vi "Main.vi"(8 "error in":errorcluster, 11 "Application Manager in":refnum<class "Application Manager.lvclass">) -> (0 "error out":errorcluster, 3 "Application Manager out":refnum<class "Application Manager.lvclass">)   [LabVIEW 2017, in "Application Manager.lvclass"]
doc: "The <b>Queued Message Handler</b> of the Worker that owns this VI."
uses:
  Application Manager.lvclass
  Buttons/Settings.ctl
  FP Refs.ctl
  <vilib>/Utility/miscctls.llb/LVPointTypeDef.ctl
  Application Manager.lvclass/Application Manager.ctl
  <vilib>/addons/_Workers/Library/Classes/Message/Priority.ctl
  Initialization Data.ctl
  Response Cases.ctl
  <vilib>/addons/_Workers/Library/Case Label.ctl
  rsp_Start Shutdown.ctl
  rql_RCM Show Message Log.ctl
  Tree Right Click Menu Data.ctl
  <vilib>/Utility/miscctls.llb/LVPoint32TypeDef.ctl
  rql_RCM Show Front Panel.ctl
  rql_RCM Show Block Diagram.ctl
  rql_RCM Send Start Exiting Request.ctl
  rql_RCM Filter as Enque Worker.ctl
  rql_RCM Filter as Deque Worker.ctl
  rwr_Get Shutdown Data Reply.ctl
  <vilib>/Utility/miscctls.llb/LVRectTypeDef.ctl
  rqp_Display User Message.ctl
  rqp_Show Front Panel.ctl
  <vilib>/Platform/browser.llb/Open URL in Default Browser (string).vi
  <vilib>/addons/_Workers/Library/Workers.lvlib
  <vilib>/addons/_Workers/Library/Classes/Message/Message.lvclass
panel:
  in  "settings":T1
  in  "ClearDisconnected":bool
  out "Message":string="Error : Port already in use"
  in  "Tree":string(tree)
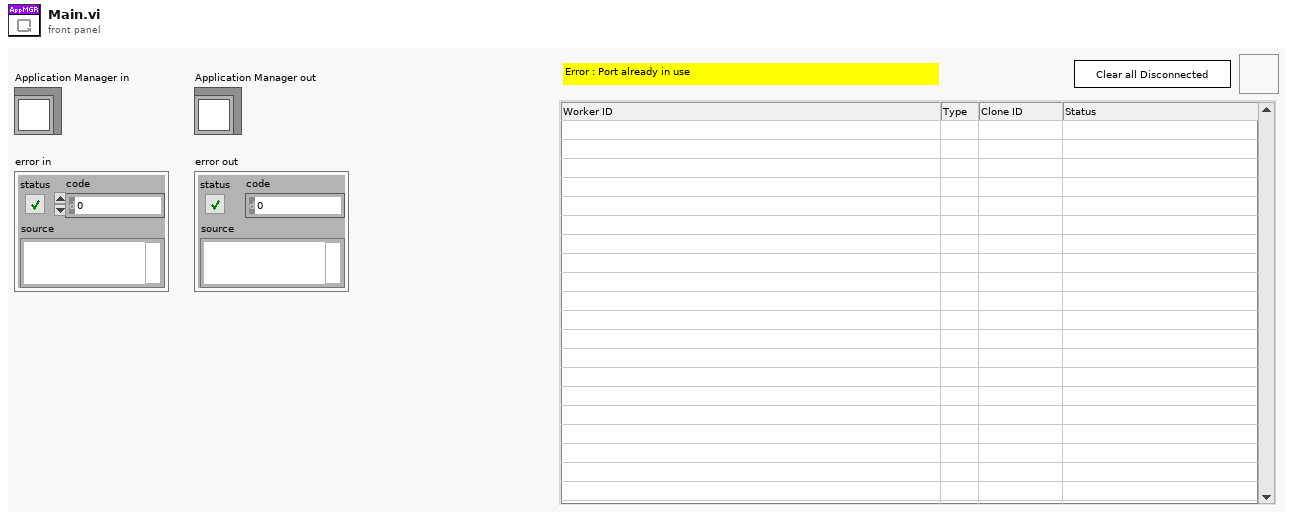
[diagram p1: front panel]
types:
  T1 = typedef "Settings.ctl" = bool
  T2 = typedef "LVPointTypeDef.ctl" = cluster{"Horizontal":i16, "Vertical":i16}
  T3 = typedef "Application Manager.lvclass/FP Refs.ctl" = cluster{"Message.Ref":refnum<vi>, "ClearDiscon.Ref":refnum<vi>, "Settings.Ref":refnum<vi>, "Tree.Ref":refnum<vi>}
  T4 = typedef "imagedata.ctl" = cluster{"image type":i32, "image depth":i32, "image":u8[], "mask":u8[], "colors":u32[], "Rectangle":cluster{"left":i16, "top":i16, "right":i16, "bottom":i16}}
  T5 = typedef "Application Manager.lvclass/Initialization Data.ctl" = cluster{"Response Cases":T6}
  T6 = typedef "Application Manager.lvclass/Response Cases.ctl" = cluster{"Show Settings Dialog":T7, "Start Shutdown":T7, "Show Message Log":T7, "New Head Worker Added":T7, "Show Worker Front Panel":T7, "Show Worker Block Diagram":T7, "Send Start Exiting Request":T7, "Filter as Enque Worker":T7, "Filter as Deque Worker":T7, "Go to MHL Case - Response":T7}
  T7 = typedef "Workers.lvlib/Case Label.ctl" = string
  T8 = typedef "Application Manager.lvclass/rsp_Start Shutdown.ctl" = cluster{"Monitor":u16}
  T9 = typedef "Workers.lvlib/Message.lvclass/Priority.ctl" = enum16{"Low", "Normal", "High"}
  T10 = typedef "Application Manager.lvclass/rql_RCM Show Message Log.ctl" = cluster{"Tree RCM Data":T11}
  T11 = typedef "Application Manager.lvclass/Tree Right Click Menu Data.ctl" = cluster{"CtlRef":refnum<vi>, "Coords":T12}
  T12 = typedef "LVPoint32TypeDef.ctl" = cluster{"Horizontal":i32, "Vertical":i32}
  T13 = typedef "Application Manager.lvclass/rql_RCM Show Front Panel.ctl" = cluster{"Tree RCM Data":T11}
  T14 = typedef "Application Manager.lvclass/rql_RCM Show Block Diagram.ctl" = cluster{"Tree RCM Data":T11}
  T15 = typedef "Application Manager.lvclass/rql_RCM Send Start Exiting Request.ctl" = cluster{"Tree RCM Data":T11}
  T16 = typedef "Application Manager.lvclass/rql_RCM Filter as Enque Worker.ctl" = cluster{"Tree RCM Data":T11}
  T17 = typedef "Application Manager.lvclass/rql_RCM Filter as Deque Worker.ctl" = cluster{"Tree RCM Data":T11}
  T18 = typedef "Application Manager.lvclass/rwr_Get Shutdown Data Reply.ctl" = cluster{"Window Bounds":T19, "Monitor":u16, "FP.State":enum32{"Invalid", "Standard", "Closed", "Hidden", "Minimized", "Maximized"}, "Column Widths":u32[]}
  T19 = typedef "LVRectTypeDef.ctl" = cluster{"Left":i16, "Top":i16, "Right":i16, "Bottom":i16}
  T20 = typedef "Application Manager.lvclass/rqp_Display User Message.ctl" = cluster{"Message":string, "BG Color":u32}
  T21 = typedef "Application Manager.lvclass/rqp_Show Front Panel.ctl" = cluster{"String":string}
  T22 = enum32{"Invalid", "Standard", "Closed", "Hidden", "Minimized", "Maximized"}
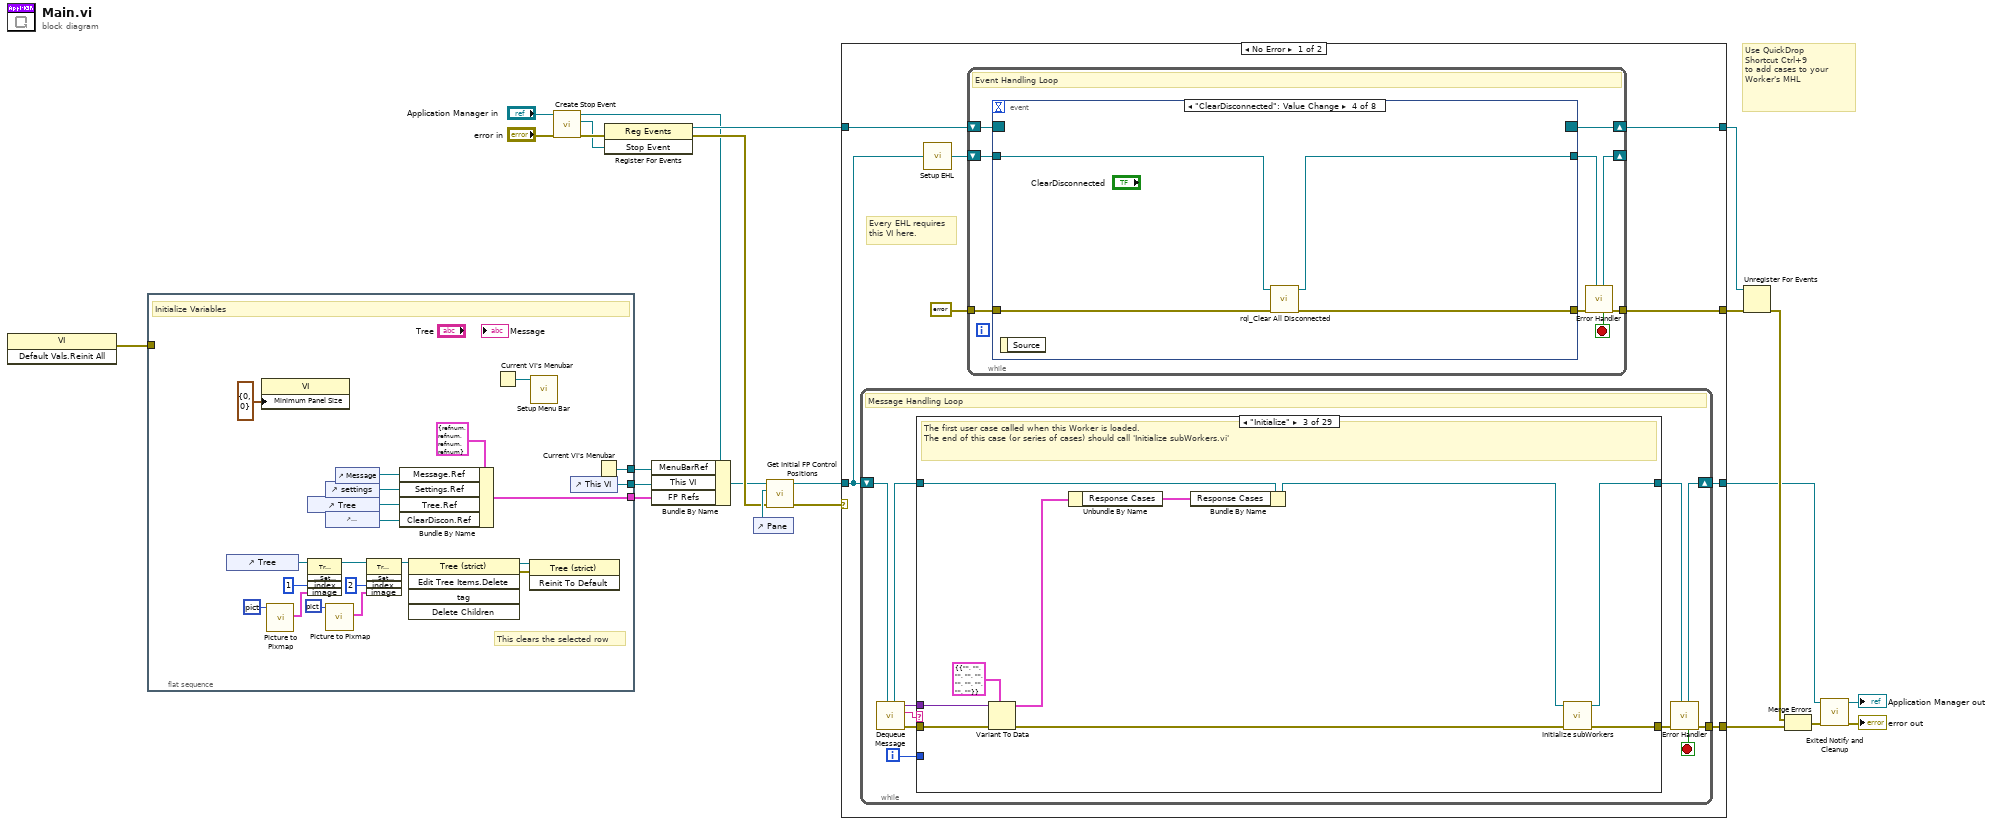
[diagram p0: block diagram]
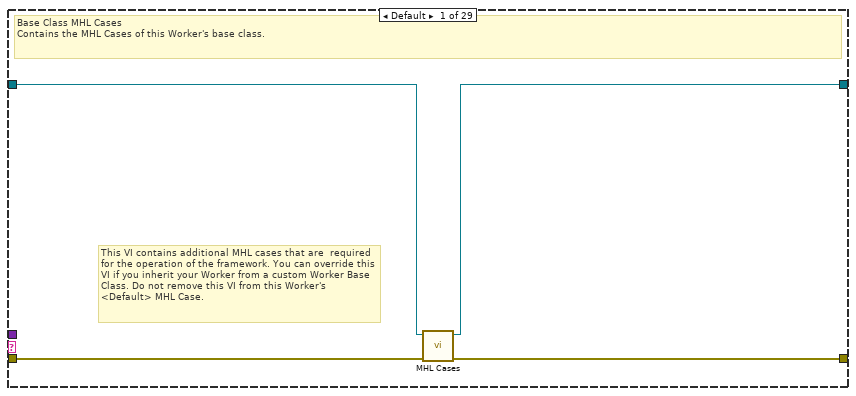
[diagram p2: hidden frame]
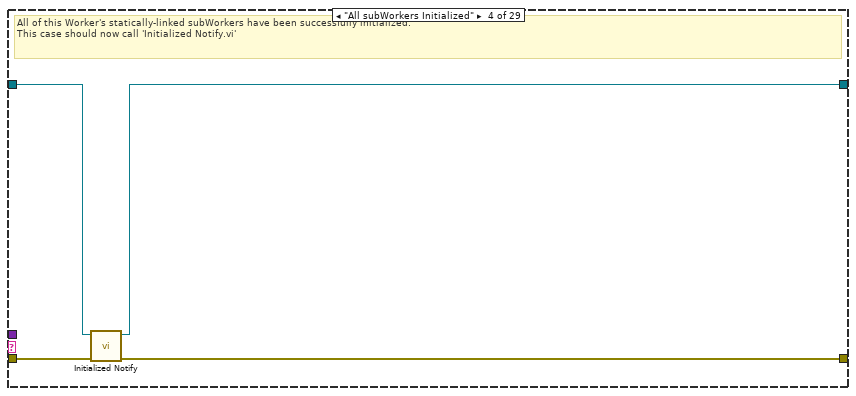
[diagram p4: hidden frame]
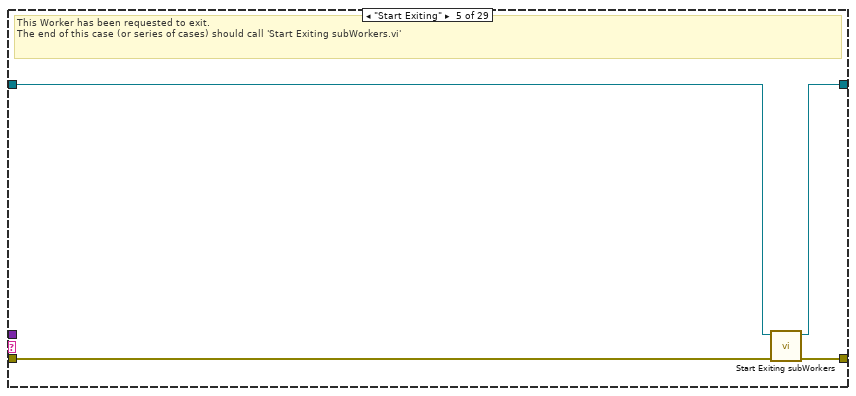
[diagram p5: hidden frame]
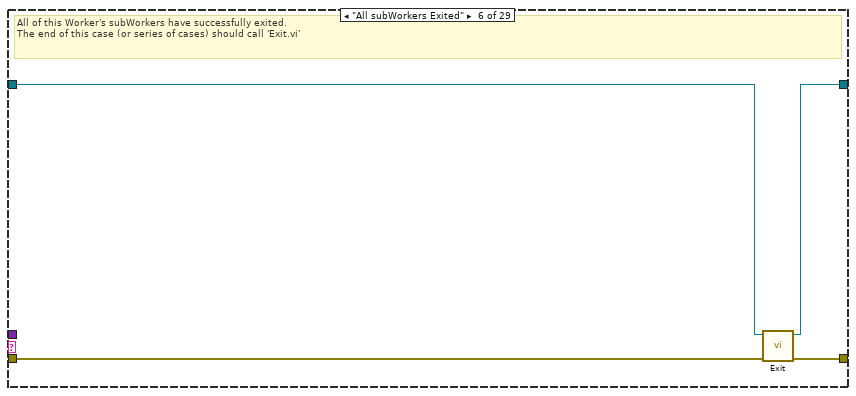
[diagram p6: hidden frame]
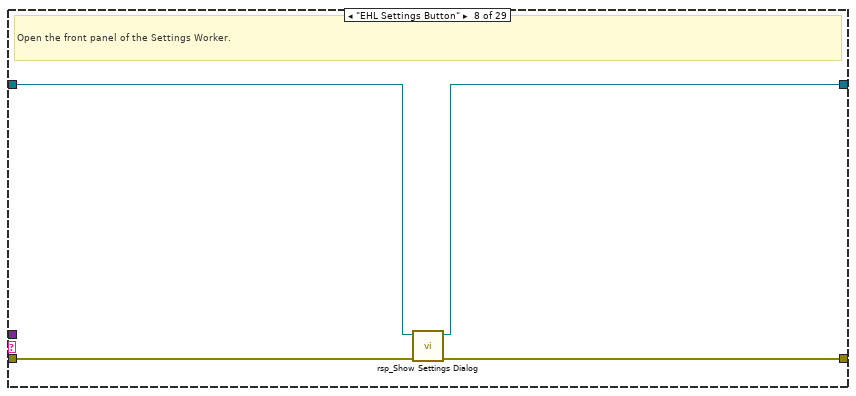
[diagram p8: hidden frame]
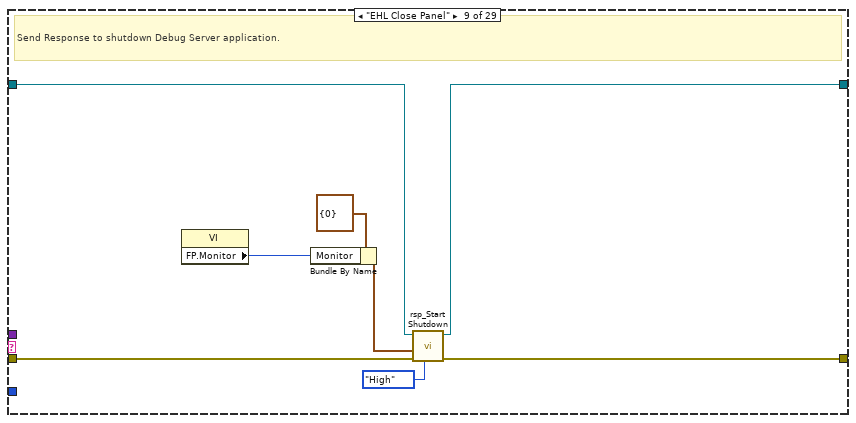
[diagram p9: hidden frame]
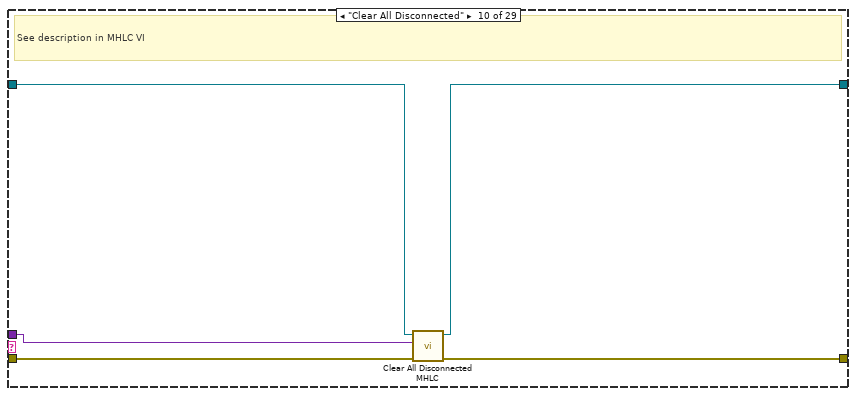
[diagram p10: hidden frame]
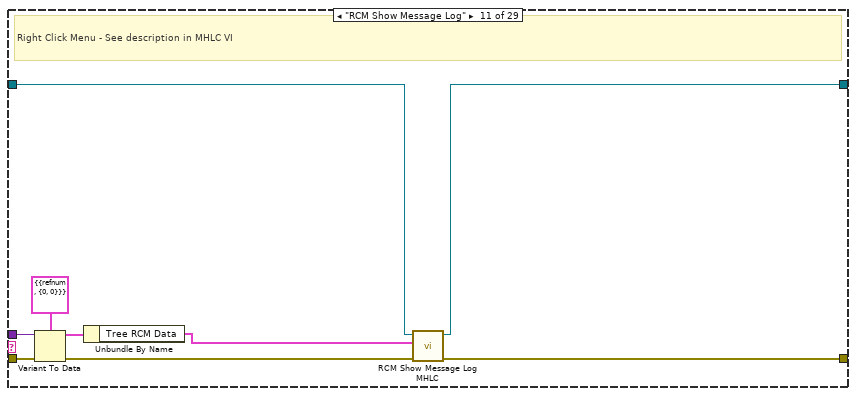
[diagram p11: hidden frame]
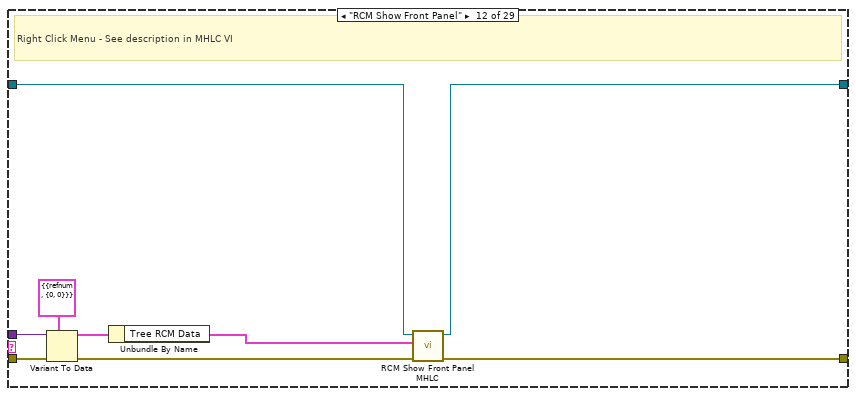
[diagram p12: hidden frame]
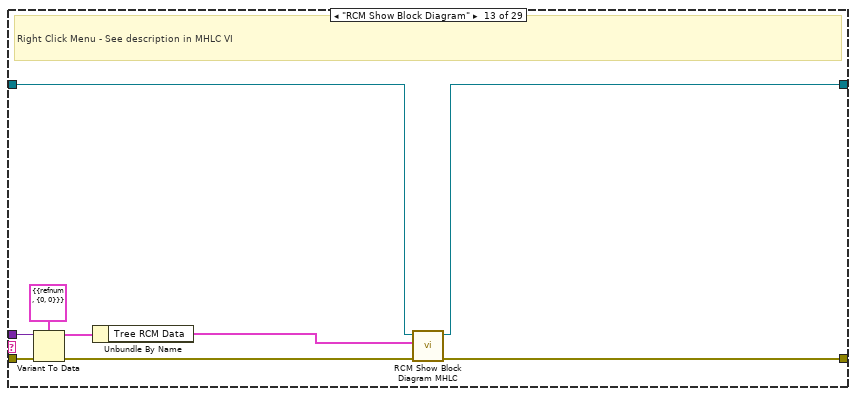
[diagram p13: hidden frame]
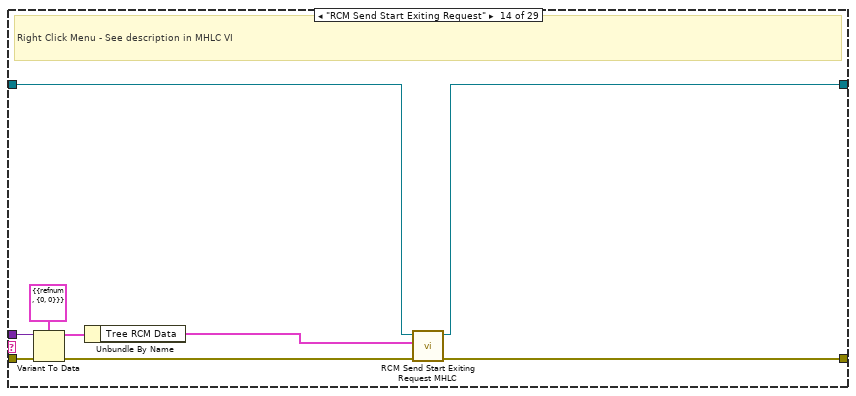
[diagram p14: hidden frame]
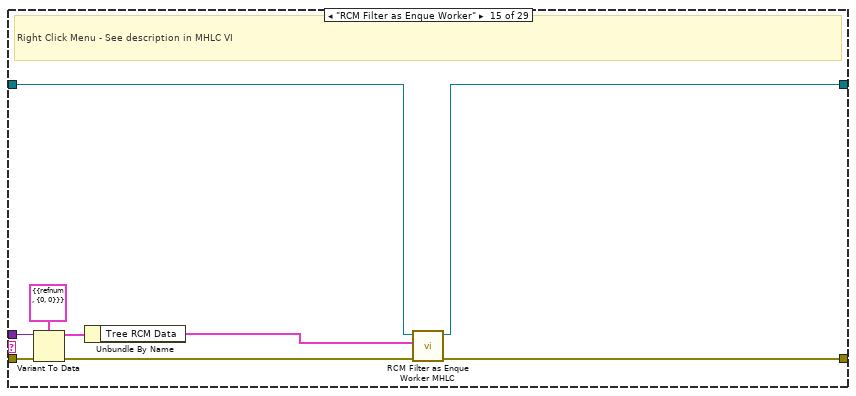
[diagram p15: hidden frame]
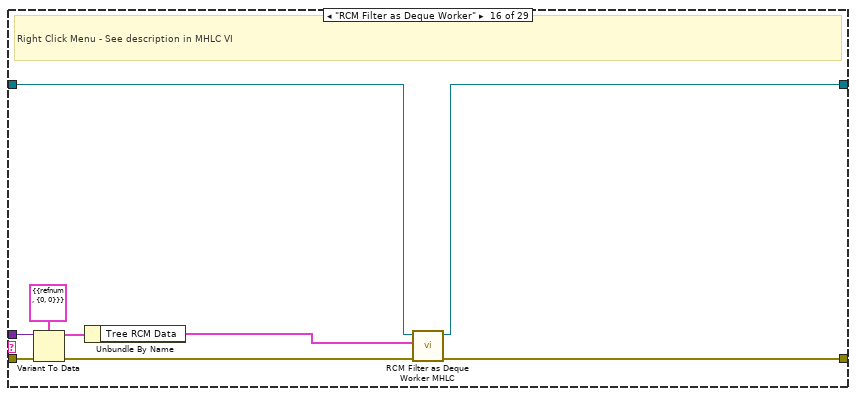
[diagram p16: hidden frame]
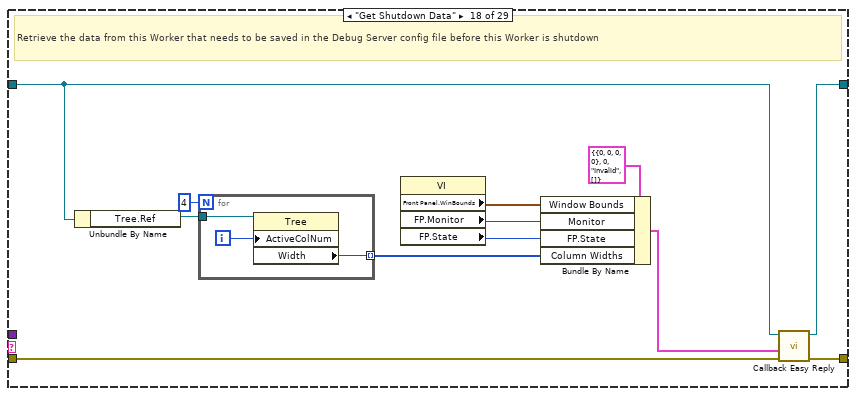
[diagram p18: hidden frame]
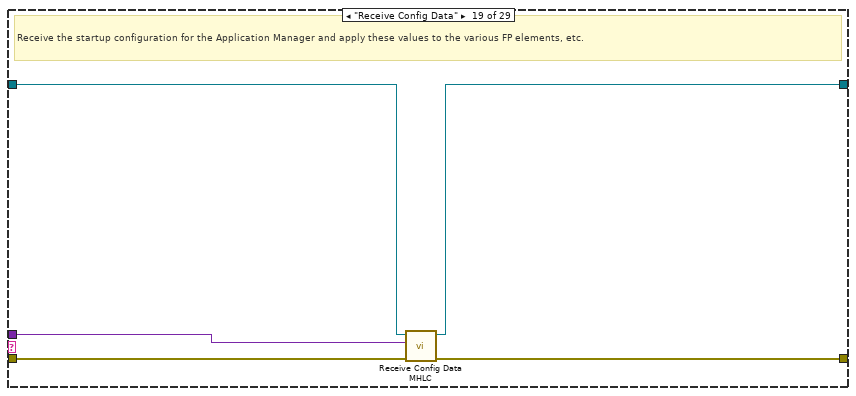
[diagram p19: hidden frame]
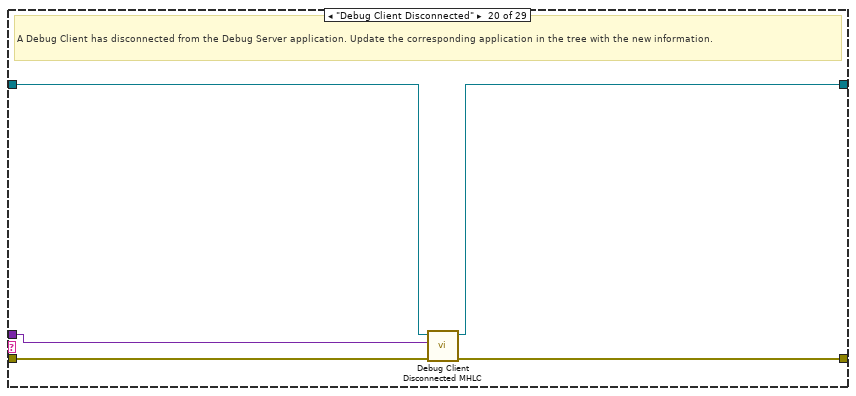
[diagram p20: hidden frame]
diagram:
  # "Use QuickDrop\nShortcut Ctrl+9\nto add cases to your\nWorker's MHL"
  n1 = invoke class="VI" method="Default Vals.Reinit All"() -> (error out=w8:errorcluster)  [unwired: 3 in, 2 out]
  n2 = flat-sequence {
    tunnel: w8 -> [_]
    tunnel: [w27] -> w5
    tunnel: [w26] -> w4
    tunnel: [w25] -> w3
    frame #0 {
      # "This clears the selected row"
      # "Initialize Variables"
      n3 = control-ref of="Tree"() -> (w33:refnum<vi>)
      n4 = property class="VI"("Minimum Panel Size"=T2 {"Horizontal"=0, "Vertical"=0} ("Front Panel Window:Minimum Size")) -> ()  [unwired: 2 in, 2 out]
      n5 = call <vilib>:"Picture to Pixmap.vi"("picture"=picture bytes[273] ("new picture")) -> ("image data"=w37:T4)  [unwired: 9 in, 1 out]
      n6 = control-ref of="Tree"() -> (w41:refnum<vi>)
      n7 = invoke on="Invoke Node" class="Tree (strict)" method="Custom Item Symbols.Set Symbol"(reference=w33, "index"=1 ("Index"), "image"=w37) -> (reference out=w38:refnum<vi>)  [unwired: 2 in, 4 out]
      n8 = control-ref of="settings"() -> (w28:refnum<vi>)
      n9 = control-ref of="ClearDisconnected"() -> (w42:refnum<vi>)
      n10 = call <vilib>:"Picture to Pixmap.vi"("picture"=picture bytes[273] ("new picture 2")) -> ("image data"=w35:T4)  [unwired: 9 in, 1 out]
      n11 = control-ref of="Message"() -> (w43:refnum<vi>)
      n12 = invoke on="Invoke Node" class="Tree (strict)" method="Custom Item Symbols.Set Symbol"(reference=w38, "index"=2 ("Index"), "image"=w35) -> (reference out=w30:refnum<vi>)  [unwired: 2 in, 4 out]
      n13 = Bundle By Name(cluster=T3 {"Message.Ref"=refnum, "ClearDiscon.Ref"=refnum, "Settings.Ref"=refnum, "Tree.Ref"=refnum} ("Data"), "Message.Ref"=w43, "Settings.Ref"=w28, "Tree.Ref"=w41, "ClearDiscon.Ref"=w42) -> (w25:T3)
      n14 = invoke class="Tree (strict)" method="Edit Tree Items.Delete"(reference=w30) -> (reference out=w32:refnum<vi>, error out=w31:errorcluster)  [unwired: 4 in, 3 out]
      n15 = Current VI's Menubar() -> (w24:refnum<k9>)
      n16 = invoke class="Tree (strict)" method="Reinit To Default"(reference=w32, error in=w31) -> ()  [unwired: 1 in, 3 out]
      n17 = call "Setup Menu Bar.vi"("menu reference"=w24) -> ()  [unwired: 10 in, 1 out]
      n18 = control-ref of="This VI"() -> (w26:refnum<vi>)
      n19 = Current VI's Menubar() -> (w27:refnum<k9>)
    }
  }
  n20 = call-dynamic "Create Stop Event.vi"("error in"="error in", "Worker"="Application Manager in") -> ("error out"=w18:errorcluster, "Stop Event"=w15:refnum<user-event>, "Worker out"=w6:refnum<class "Application Manager.lvclass">)  [unwired: 7 in]
  n21 = register-events(error in=w18, w15) -> (reference out=w17:refnum<event-registration>, error out=w9:errorcluster)  [unwired: 1 in]
  n22 = Bundle By Name(cluster=w6, "MenuBarRef"=w5, "This VI"=w4, "FP Refs"=w3) -> (w7:refnum<class "Application Manager.lvclass">)
  n23 = control-ref of="Pane"() -> (w10:refnum<vi>)
  n24 = call "Get Initial FP Control Positions.vi"("error in (no error)"=w9, "Pane"=w10, "AppMgr in"=w7) -> ("error out"=w2:errorcluster, "AppMgr out"=w1:refnum<class "Application Manager.lvclass">)  [unwired: 7 in]
  n25 = case shown="No Error" w2 {
    tunnel: w1 -> [w47 w309]
    tunnel: [w45 w310] -> w16
    tunnel: w17 -> [w52 w311]
    tunnel: [w49 w312] -> w22
    tunnel: [w51 w311] -> w21
    tunnel: [w46 w308] -> w19
    selector: w2 -> [_ w312]
    frame No Error {
      # "Every EHL requires\nthis VI here."
      n26 = while {
        shift-right: [w61] -> w46
        shift-left: w47 -> [w63]
        tunnel: [w62] -> w45
        i -> [w54]
        stop <- w55 stop-if-true
        # "Message Handling Loop"
        n27 = call-dynamic "Dequeue Message.vi"("Worker"=w63) -> ("error out"=w60:errorcluster, "Case out"=w56:string, "Data out"=w53:variant, "Worker out"=w58:refnum<class "Application Manager.lvclass">)  [unwired: 6 in, 1 out]
        n28 = case "Worker MHL Case Structure (DO NOT CHANGE LABEL NAME)" shown="\"Initialize\"" w56 {
          tunnel: w60 -> [w67 w68 w77 w81 w84 w91 w93 w97 w105 w110 w114 w128 w137 w146 w155 w164 w166 w178 w186 w191 w202 w208 w213 w218 w220 w225 w230 w235 w240]
          tunnel: [w66 w68 w79 w80 w87 w90 w93 w96 w104 w109 w119 w127 w132 w141 w150 w159 w166 w177 w182 w189 w201 w206 w210 w217 w220 w223 w229 w234 w239] -> w59
          tunnel: w58 -> [w65 w69 w76 w83 w85 w89 w92 w95 w103 w108 w118 w126 w131 w140 w149 w158 w165 w168 w185 w188 w197 w207 w211 w216 w219 w222 w228 w233 w238]
          tunnel: [w64 w69 w78 w82 w86 w88 w92 w94 w102 w107 w117 w125 w130 w139 w148 w157 w165 w176 w184 w187 w197 w207 w209 w215 w219 w221 w227 w232 w237] -> w57
          tunnel: w54 -> [_ _ _ _ _ _ _ _ _ _ _ _ _ _ _ _ _ _ _ _ _ _ _ _ _ _ _ _ _]
          tunnel: w53 -> [_ _ w74 _ _ _ _ _ _ w106 w115 w123 w134 w143 w152 w161 _ _ w183 w190 w199 w204 w212 w214 _ w224 w226 w231 w236]
          frame Default {
            # "This VI contains additional MHL cases that are  required for the operation of the framework. You can override this VI if you inherit your Worker from a custom Worker Base Class. Do not remove this VI from this Worker's <Default> MHL Case."
            # "Base Class MHL Cases\nContains the MHL Cases of this Worker's base class."
            n29 = call-dynamic "MHL Cases.vi"("error in"=w67, "Worker in"=w65) -> ("error out"=w66:errorcluster, "Worker out"=w64:refnum<class "Application Manager.lvclass">)  [unwired: 8 in]
          }
          frame "------------ FRAMEWORK CASES -----------" {
            # "Start of Workers Framework Cases"
          }
          frame "Initialize" {
            # "The first user case called when this Worker is loaded.\nThe end of this case (or series of cases) should call 'Initialize subWorkers.vi'"
            n30 = Variant To Data(error in=w77, type=T5 {"Response Cases"={"Show Settings Dialog"="", "Start Shutdown"="", "Show Message Log"="", "New Head Worker Added"="", "Show Worker Front Panel"="", "Show Worker Block Diagram"="", "Send Start Exiting Request"="", "Filter as Enque Worker"="", "Filter as Deque Worker"="", "Go to MHL Case - Response"=""}} ("Initialization Data"), Variant=w74) -> (data=w71:T5, error out=w75:errorcluster)
            n31 = Unbundle By Name(w71) -> ("Response Cases"=w70:T6)
            n32 = Bundle By Name(cluster=w76, "Response Cases"=w70) -> (w72:refnum<class "Application Manager.lvclass">)
            n33 = call-dynamic "Initialize subWorkers.vi"("error in"=w75, "Worker"=w72) -> ("error out"=w79:errorcluster, "dup Worker out"=w78:refnum<class "Application Manager.lvclass">)  [unwired: 8 in]
          }
          frame "All subWorkers Initialized" {
            # "All of this Worker's statically-linked subWorkers have been successfully initialized.\nThis case should now call 'Initialized Notify.vi'"
            n34 = call-dynamic "Initialized Notify.vi"("error in"=w81, "Worker"=w83) -> ("error out"=w80:errorcluster, "dup Worker out"=w82:refnum<class "Application Manager.lvclass">)  [unwired: 8 in]
          }
          frame "Start Exiting" {
            # "This Worker has been requested to exit. \nThe end of this case (or series of cases) should call 'Start Exiting subWorkers.vi'"
            n35 = call-dynamic "Start Exiting subWorkers.vi"("error_in"=w84, "Worker"=w85) -> ("error out"=w87:errorcluster, "dup Worker out"=w86:refnum<class "Application Manager.lvclass">)  [unwired: 8 in]
          }
          frame "All subWorkers Exited" {
            # "All of this Worker's subWorkers have successfully exited. \nThe end of this case (or series of cases) should call 'Exit.vi'"
            n36 = call-dynamic "Exit.vi"("error_in"=w91, "Worker"=w89) -> ("error out"=w90:errorcluster, "dup Worker out"=w88:refnum<class "Application Manager.lvclass">)  [unwired: 8 in]
          }
          frame "------------- LOCAL API CASES -------------" {
            # "Start of Workers Local API Cases"
          }
          frame "EHL Settings Button" {
            # "Open the front panel of the Settings Worker."
            n37 = call "rsp_Show Settings Dialog.vi"("error in"=w97, "Application Manager in"=w95) -> ("error out"=w96:errorcluster, "dup Application Manager out"=w94:refnum<class "Application Manager.lvclass">)  [unwired: 8 in]
          }
          frame "EHL Close Panel" {
            # "Send Response to shutdown Debug Server application."
            n38 = property class="VI"() -> ("FP.Monitor"=w98:u16)  [unwired: 2 in, 2 out]
            n39 = Bundle By Name(cluster=T8 {"Monitor"=0} ("Data in"), "Monitor"=w98) -> (w99:T8)
            n40 = call "rsp_Start Shutdown.vi"("Message Priority"=Priority."High", "error in"=w105, "Data in"=w99, "Application Manager in"=w103) -> ("error out"=w104:errorcluster, "dup Application Manager out"=w102:refnum<class "Application Manager.lvclass">)  [unwired: 6 in]
          }
          frame "Clear All Disconnected" {
            # "See description in MHLC VI"
            n41 = call "Clear All Disconnected MHLC.vi"("error in (no error)"=w110, "Data in"=w106, "AppMgr in"=w108) -> ("error out"=w109:errorcluster, "AppMgr out"=w107:refnum<class "Application Manager.lvclass">)  [unwired: 7 in]
          }
          frame "RCM Show Message Log" {
            # "Right Click Menu - See description in MHLC VI"
            n42 = Variant To Data(error in=w114, type=T10 {"Tree RCM Data"={"CtlRef"=refnum, "Coords"={"Horizontal"=0, "Vertical"=0}}} ("Data"), Variant=w115) -> (data=w112:T10, error out=w113:errorcluster)
            n43 = Unbundle By Name(w112) -> ("Tree RCM Data"=w111:T11)
            n44 = call "RCM Show Message Log MHLC.vi"("error in (no error)"=w113, "Tree RCM Data"=w111, "AppMgr in"=w118) -> ("error out"=w119:errorcluster, "AppMgr out"=w117:refnum<class "Application Manager.lvclass">)  [unwired: 7 in]
          }
          frame "RCM Show Front Panel" {
            # "Right Click Menu - See description in MHLC VI"
            n45 = Variant To Data(error in=w128, type=T13 {"Tree RCM Data"={"CtlRef"=refnum, "Coords"={"Horizontal"=0, "Vertical"=0}}} ("Data"), Variant=w123) -> (data=w121:T13, error out=w124:errorcluster)
            n46 = Unbundle By Name(w121) -> ("Tree RCM Data"=w120:T11)
            n47 = call "RCM Show Front Panel MHLC.vi"("error in (no error)"=w124, "Tree RCM Data"=w120, "AppMgr in"=w126) -> ("error out"=w127:errorcluster, "AppMgr out"=w125:refnum<class "Application Manager.lvclass">)  [unwired: 7 in]
          }
          frame "RCM Show Block Diagram" {
            # "Right Click Menu - See description in MHLC VI"
            n48 = Variant To Data(error in=w137, type=T14 {"Tree RCM Data"={"CtlRef"=refnum, "Coords"={"Horizontal"=0, "Vertical"=0}}} ("Data"), Variant=w134) -> (data=w133:T14, error out=w136:errorcluster)
            n49 = Unbundle By Name(w133) -> ("Tree RCM Data"=w129:T11)
            n50 = call "RCM Show Block Diagram MHLC.vi"("error in (no error)"=w136, "Tree RCM Data"=w129, "AppMgr in"=w131) -> ("error out"=w132:errorcluster, "AppMgr out"=w130:refnum<class "Application Manager.lvclass">)  [unwired: 7 in]
          }
          frame "RCM Send Start Exiting Request" {
            # "Right Click Menu - See description in MHLC VI"
            n51 = Variant To Data(error in=w146, type=T15 {"Tree RCM Data"={"CtlRef"=refnum, "Coords"={"Horizontal"=0, "Vertical"=0}}} ("Data"), Variant=w143) -> (data=w142:T15, error out=w145:errorcluster)
            n52 = Unbundle By Name(w142) -> ("Tree RCM Data"=w138:T11)
            n53 = call "RCM Send Start Exiting Request MHLC.vi"("error in (no error)"=w145, "Tree RCM Data"=w138, "AppMgr in"=w140) -> ("error out"=w141:errorcluster, "AppMgr out"=w139:refnum<class "Application Manager.lvclass">)  [unwired: 7 in]
          }
          frame "RCM Filter as Enque Worker" {
            # "Right Click Menu - See description in MHLC VI"
            n54 = Variant To Data(error in=w155, type=T16 {"Tree RCM Data"={"CtlRef"=refnum, "Coords"={"Horizontal"=0, "Vertical"=0}}} ("Data"), Variant=w152) -> (data=w151:T16, error out=w154:errorcluster)
            n55 = Unbundle By Name(w151) -> ("Tree RCM Data"=w147:T11)
            n56 = call "RCM Filter as Enque Worker MHLC.vi"("error in (no error)"=w154, "Tree RCM Data"=w147, "AppMgr in"=w149) -> ("error out"=w150:errorcluster, "AppMgr out"=w148:refnum<class "Application Manager.lvclass">)  [unwired: 7 in]
          }
          frame "RCM Filter as Deque Worker" {
            # "Right Click Menu - See description in MHLC VI"
            n57 = Variant To Data(error in=w164, type=T17 {"Tree RCM Data"={"CtlRef"=refnum, "Coords"={"Horizontal"=0, "Vertical"=0}}} ("Data"), Variant=w161) -> (data=w160:T17, error out=w163:errorcluster)
            n58 = Unbundle By Name(w160) -> ("Tree RCM Data"=w156:T11)
            n59 = call "RCM Filter as Deque Worker MHLC.vi"("error in (no error)"=w163, "Tree RCM Data"=w156, "AppMgr in"=w158) -> ("error out"=w159:errorcluster, "AppMgr out"=w157:refnum<class "Application Manager.lvclass">)  [unwired: 7 in]
          }
          frame "------------- PUBLIC API CASES -------------" {
            # "Start of Workers Public API Cases"
          }
          frame "Get Shutdown Data" {
            # "Retrieve the data from this Worker that needs to be saved in the Debug Server config file before this Worker is shutdown"
            n60 = Unbundle By Name(w168) -> ("Tree.Ref"=w167:refnum<vi>)
            n61 = for {
              N: 4 -> [_]
              tunnel: [w181] -> w169 mode=indexing
              tunnel: w167 -> [w179]
              i -> [w180]
              n62 = property class="Tree"(reference=w179, "ActiveColNum"=w180) -> ("Width"=w181:i32)  [unwired: 1 in, 2 out]
            }
            n63 = property class="VI"() -> ("Front Panel.WinBounds"=w173:T19, "FP.Monitor"=w172:u16, "FP.State"=w171:T22)  [unwired: 2 in, 2 out]
            n64 = Bundle By Name(cluster=T18 {"Window Bounds"={"Left"=0, "Top"=0, "Right"=0, "Bottom"=0}, "Monitor"=0, "FP.State"=enum."Invalid", "Column Widths"=[]} ("Reply Data"), "Window Bounds"=w173, "Monitor"=w172, "FP.State"=w171, "Column Widths"=w169) -> (w174:T18)
            n65 = call-dynamic "Callback Easy Reply.vi"("error in"=w178, "Data"=w174, "Worker"=w168) -> ("error out"=w177:errorcluster, "dup Worker out"=w176:refnum<class "Application Manager.lvclass">)  [unwired: 7 in]
          }
          frame "Receive Config Data" {
            # "Receive the startup configuration for the Application Manager and apply these values to the various FP elements, etc."
            n66 = call "Receive Config Data MHLC.vi"("error in (no error)"=w186, "Data"=w183, "AppMgr in"=w185) -> ("error out"=w182:errorcluster, "AppMgr out"=w184:refnum<class "Application Manager.lvclass">)  [unwired: 7 in]
          }
          frame "Debug Client Disconnected" {
            # "A Debug Client has disconnected from the Debug Server application. Update the corresponding application in the tree with the new information."
            n67 = call "Debug Client Disconnected MHLC.vi"("error in (no error)"=w191, "Data in"=w190, "AppMgr in"=w188) -> ("error out"=w189:errorcluster, "AppMgr out"=w187:refnum<class "Application Manager.lvclass">)  [unwired: 7 in]
          }
          frame "Display User Message" {
            # "Update the User Message string with the new status"
            n68 = Variant To Data(error in=w202, type=T20 {"Message"="", "BG Color"=0} ("Data"), Variant=w199) -> (data=w198:T20, error out=w201:errorcluster)
            n69 = Unbundle By Name(w198) -> ("Message"=w195:string, "BG Color"=w194:u32)
            n70 = Unbundle By Name(w197) -> ("Message.Ref"=w196:refnum<vi>)
            n71 = Concatenate Strings("Status : " ("string"), w195) -> (w193:string)
            n72 = property class="Str"(reference=w196, "Value"=w193, "Text.BGColor"=w194) -> ()  [unwired: 1 in, 2 out]
          }
          frame "Show Front Panel" {
            # "Show the front panel of the Application Manager"
            n73 = Variant To Data(error in=w208, type=T21 {"String"=""} ("Data"), Variant=w204) -> (data=w203:T21, error out=w206:errorcluster)
            n74 = Unbundle By Name(w203) -> ()  [unwired: 1 out]
            n75 = invoke class="VI" method="FP.Open"() -> ()  [unwired: 5 in, 5 out]
          }
          frame "Open Running VI" {
            # "Open the Front Panel of the Main VI of the selected Worker's running clone"
            n76 = call "Open Running VI MHLC.vi"("error in (no error)"=w213, "Data in"=w212, "AppMgr in"=w211) -> ("error out"=w210:errorcluster, "AppMgr out"=w209:refnum<class "Application Manager.lvclass">)  [unwired: 7 in]
          }
          frame "Go to MHL Case" {
            # "Show the selected MHL on the block diagram of the Main VI of the selected Worker"
            n77 = call "Go to MHL Case MHLC.vi"("error in (no error)"=w218, "Data in"=w214, "AppMgr in"=w216) -> ("error out"=w217:errorcluster, "AppMgr out"=w215:refnum<class "Application Manager.lvclass">)  [unwired: 7 in]
          }
          frame "----------- DEBUG CLIENT CASES ------------" {
            # "These cases are called externally by the Debug Client application\nMessages are forwarded to these cases directly by the DS TCP Read Worker"
          }
          frame "Add New Worker" {
            # "Sent from Normal priority read Worker"
            # "See description in MHLC VI"
            n78 = call "Add New Worker MHLC.vi"("error in (no error)"=w225, "Data in"=w224, "AppMgr in"=w222) -> ("error out"=w223:errorcluster, "AppMgr out"=w221:refnum<class "Application Manager.lvclass">)  [unwired: 7 in]
          }
          frame "Add Worker VI Ref" {
            # "Sent from Normal priority read Worker"
            # "See description in MHLC VI"
            n79 = call "Add Worker VI Ref MHLC.vi"("error in (no error)"=w230, "Data in"=w226, "AppMgr in"=w228) -> ("error out"=w229:errorcluster, "AppMgr out"=w227:refnum<class "Application Manager.lvclass">)  [unwired: 7 in]
          }
          frame "Update Worker Status" {
            # "Sent from Normal priority read Worker"
            # "See description in MHLC VI"
            n80 = call "Update Worker Status MHLC.vi"("error in (no error)"=w235, "Data in"=w231, "AppMgr in"=w233) -> ("error out"=w234:errorcluster, "AppMgr out"=w232:refnum<class "Application Manager.lvclass">)  [unwired: 7 in]
          }
          frame "Application Aborted" {
            # "Sent from Normal priority read Worker"
            # "See description in MHLC VI"
            n81 = call "Application Aborted MHLC.vi"("error in (no error)"=w240, "Data in"=w236, "AppMgr in"=w238) -> ("error out"=w239:errorcluster, "AppMgr out"=w237:refnum<class "Application Manager.lvclass">)  [unwired: 7 in]
          }
        }
        n82 = call-dynamic "Error Handler.vi"("Worker"=w57, "error_in"=w59) -> ("error out"=w62:errorcluster, "Stop Loop"=w55:bool, "Worker out"=w61:refnum<class "Application Manager.lvclass">)  [unwired: 7 in]
      }
      n83 = call-dynamic "Setup EHL.vi"("Worker"=w47) -> ("Worker out"=w48:refnum<class "Application Manager.lvclass">)  [unwired: 14 in]
      n84 = while "Event Handling Loop" {
        shift-right: [w249] -> w51
        shift-left: w52 -> [w248]
        tunnel: [w244] -> w49
        tunnel: errorcluster {"status"=FALSE, "code"=0, "source"=""} ("error constant") -> [w246]
        shift-right: [w242] -> _
        shift-left: w48 -> [w247]
        stop <- w241 stop-if-true
        # "Event Handling Loop"
        n85 = event shown="[3] \"ClearDisconnected\": Value Change" {
          selector: w248 -> [_ _ _ _ _ _ _ _]
          dyn-events: [_ _ _ _ _ _ _ _] -> w249
          timeout: _ -> [_ _ _ _ _ _ _ _]
          tunnel: [w253 w258 w264 w283 w287 w289 w301 w306] -> w245
          tunnel: w246 -> [w254 w259 w265 w284 w288 w291 w302 w307]
          tunnel: w247 -> [w252 w257 w263 w282 w286 w295 w300 w305]
          tunnel: [w251 w256 w262 w281 w285 w295 w299 w304] -> w243
          event User Event {
            # "This case and its contents must always be included in every EHL that you use, so that the framework can automatically stop the EHL."
            # "EHL Stop Event. This EHL exits from this case."
            n86 = event-data() -> ("Stop Event Data"=w250:variant)  [unwired: 1 in]
            n87 = call-dynamic "EHL Stop - EHL Case.vi"("error in"=w254, "Stop Event Data"=w250, "Worker"=w252) -> ("error out"=w253:errorcluster, "Worker out"=w251:refnum<class "Application Manager.lvclass">)  [unwired: 7 in]
          }
          event Panel Close? {
            # "Calls the Start Exiting case of this Worker. This will start the exiting sequence of this Worker."
            n88 = event-data() -> ()  [unwired: 1 in, 1 out]
            n89 = call "rql_EHL Close Panel.vi"("Message Priority"=Priority."High", "error in"=w259, "Application Manager in"=w257) -> ("error out"=w258:errorcluster, "dup Application Manager out"=w256:refnum<class "Application Manager.lvclass">)  [unwired: 7 in]
            n90 = event-data("Discard?"=TRUE) -> ()  [unwired: 1 in, 1 out]
          }
          event Menu Selection (User) {
            n91 = event-data() -> ("ItemTag"=w261:string)  [unwired: 1 in]
            n92 = case shown="\"Exit\"" w261 {
              tunnel: w265 -> [w266 w272 w274 w277 w280]
              tunnel: [w266 w271 w273 w277 w280] -> w264
              tunnel: w263 -> [w267 w270 w275 w278 w279]
              tunnel: [w267 w269 w275 w278 w279] -> w262
              frame Default {
              }
              frame "Exit" {
                n93 = call "rql_EHL Close Panel.vi"("Message Priority"=Priority."High", "error in"=w272, "Application Manager in"=w270) -> ("error out"=w271:errorcluster, "dup Application Manager out"=w269:refnum<class "Application Manager.lvclass">)  [unwired: 7 in]
              }
              frame "Workers 4.0 Debug Server" {
                n94 = call "Workers 4.0 Debug Server EXE Launcher.vi"("error in (no error)"=w274) -> ("error out"=w273:errorcluster)  [unwired: 10 in]
              }
              frame "Online Help" {
                n95 = call-poly <vilib>:"Open URL in Default Browser.vi"("URL"="https://docs.workersforlabview.io/v/5.0/workers-tools/workers-tools-menu/workers-debug-server/workers-application-manager") -> ()  [unwired: 5 in, 2 out]
              }
              frame "About" {
                n96 = call "About Dialog.vi"() -> ()  [unwired: 12 in]
              }
            }
          }
          event "ClearDisconnected": Value Change {
            n97 = event-data() -> ()  [unwired: 1 in, 1 out]
            n98 = call "rql_Clear All Disconnected.vi"("error in"=w284, "Application Manager in"=w282) -> ("error out"=w283:errorcluster, "dup Application Manager out"=w281:refnum<class "Application Manager.lvclass">)  [unwired: 8 in]
          }
          event Value Change {
            n99 = event-data() -> ()  [unwired: 1 in, 1 out]
            n100 = call "rql_EHL Settings Button.vi"("error in"=w288, "Application Manager in"=w286) -> ("error out"=w287:errorcluster, "dup Application Manager out"=w285:refnum<class "Application Manager.lvclass">)  [unwired: 8 in]
          }
          event "Tree": Shortcut Menu Activation? {
            w294 = string[] ["Show Message Log", "app_separator", "Show Front Panel", "Show Block Diagram", "Send 'Start Exiting' Request", "app_separator", "Filter as Enque Worker", "Filter as Deque Worker"] ("item names")
            # "The menu items are hardcoded here\nbecause VIPM loses track of the link\nto the .rtm file (if one is used)"
            n101 = event-data() -> ("MenuRef"=w290:refnum<k9>)  [unwired: 1 in]
            n102 = Delete Menu Items(6:w291, 9:w290) -> (0:w293:errorcluster, 3:w292:refnum<k9>)  [unwired: 2 in]
            n103 = Insert Menu Items(6:w293, 7:w294, 8:w294, 9:w292) -> (0:w289:errorcluster)  [unwired: 2 in, 2 out]
            n104 = event-data() -> ()  [unwired: 2 in, 1 out]
          }
          event "Tree": Shortcut Menu Selection (User) {
            n105 = event-data() -> ("CtlRef"=w298:refnum<vi>, "Coords"=w297:T12, "ItemPath"=w296:string)  [unwired: 1 in]
            n106 = call "Tree Shortcut Menu Selection.vi"("ItemPath"=w296, "error in (no error)"=w302, "Coords"=w297, "CtlRef"=w298, "AppMgr in"=w300) -> ("error out"=w301:errorcluster, "AppMgr out"=w299:refnum<class "Application Manager.lvclass">)  [unwired: 5 in]
          }
          event Pane Size {
            n107 = event-data() -> ()  [unwired: 1 in, 1 out]
            n108 = control-ref of="Pane"() -> (w303:refnum<vi>)
            n109 = call "Scale FP Controls.vi"("error in (no error)"=w307, "Pane"=w303, "AppMgr in"=w305) -> ("error out"=w306:errorcluster, "AppMgr out"=w304:refnum<class "Application Manager.lvclass">)  [unwired: 7 in]
          }
        }
        n110 = call-dynamic "Error Handler.vi"("Worker"=w243, "error_in"=w245) -> ("error out"=w244:errorcluster, "Stop Loop"=w241:bool, "Worker out"=w242:refnum<class "Application Manager.lvclass">)  [unwired: 7 in]
      }
    }
    frame Error {
      n111 = call-dynamic "Error Handler.vi"("Worker"=w309, "error_in"=w312) -> ("error out"=w310:errorcluster, "Worker out"=w308:refnum<class "Application Manager.lvclass">)  [unwired: 7 in, 1 out]
    }
  }
  n112 = Unregister For Events(event registration refnum=w21, error in=w22) -> (error out=w23:errorcluster)
  n113 = Merge Errors(w23, w16) -> (w20:errorcluster)
  n114 = call-dynamic "Exited Notify and Cleanup.vi"("error_in"=w20, "Worker"=w19) -> ("error out"=→"error out":errorcluster, "dup Worker out"=→"Application Manager out":refnum<class "Application Manager.lvclass">)  [unwired: 8 in]
